vi "Main.vi"() -> ()   [LabVIEW 2009]
panel:
  in  "Colors":T1={"False state Button color"=16118498, "True state  Button color"=10983021, "Focused color"=12826781, "Decoration Color"=2098432}
  in  "Buttons name":T2={"Caption.button0"="Starts the test sequence", "Button.name0"="Measure", "Caption.button1"="Cross correlation", "Button.name1"="Analyze", "Caption.button2"="Prints the test data report", "Button.name2"="Present", "Caption.button3"="Quits the application", "Button.name3"="Exit"}
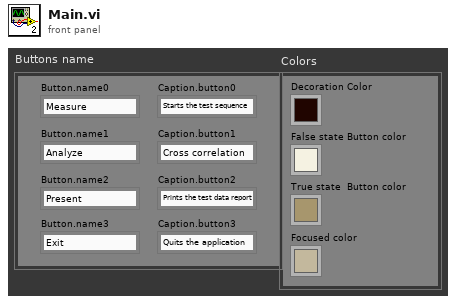
[diagram p1: front panel]
types:
  T1 = cluster{"False state Button color":u32, "True state  Button color":u32, "Focused color":u32, "Decoration Color":u32}
  T2 = cluster{"Caption.button0":string, "Button.name0":string, "Caption.button1":string, "Button.name1":string, "Caption.button2":string, "Button.name2":string, "Caption.button3":string, "Button.name3":string}
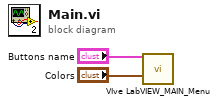
[diagram p0: block diagram]
diagram:
  n1 = call "VIve LabVIEW_MAIN_Menu.vi"("Buttons name"="Buttons name", "Colors"="Colors") -> ()  [unwired: 11 in, 3 out]
